vi "Initialize.vi"(8 "error in (no error)":errorcluster, 11 "socket REQ in":refnum<class "socket REQ.lvclass">) -> (0 "error out":errorcluster, 3 "socket REQ out":refnum<class "socket REQ.lvclass">)   [LabVIEW 2018, in "socket REQ.lvclass"]
uses:
  socket REQ.lvclass
  C:/Users/devstaff/sparc4/s4gui/Versao ZeroMQ REQ-REP/SPARC4_GUI -v1.0.8 - com pacote communication manager/communication-manager/Socket/Socket.lvclass
  Socket/Socket.lvclass
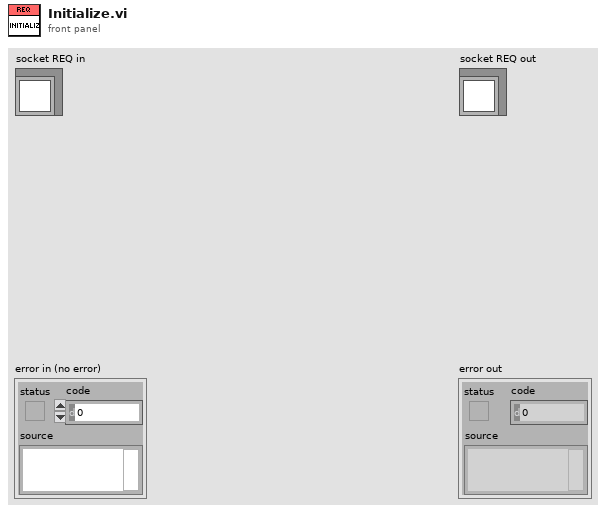
[diagram p1: front panel]
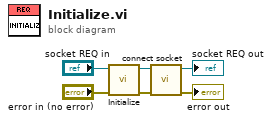
[diagram p0: block diagram]
diagram:
  n1 = call-parent "Initialize.vi"("error in (no error)"="error in (no error)", "Socket in"="socket REQ in") -> ("error out"=w3:errorcluster, "Socket out"=w4:refnum<class "socket REQ.lvclass">)  [unwired: 8 in]
  n2 = call "connect socket.vi"("error in (no error)"=w3, "Socket in"=w4) -> ("error out"=→"error out":errorcluster, "Socket out"=→"socket REQ out":refnum<class "socket REQ.lvclass">)  [unwired: 8 in]
